vi "Test 4_5.vi"(8 "error in (no error)":errorcluster, 11 "Test Case In":refnum<class "Tests.lvclass">) -> (0 "error out":errorcluster, 3 "Test Case Out":refnum<class "Tests.lvclass">)   [LabVIEW 2021, in "Tests.lvclass"]
uses:
  Tests.lvclass
  C:/Program Files (x86)/National Instruments/LabVIEW 2021/vi.lib/Astemes/LUnit/Test Case.lvclass
  <vilib>/Astemes/LUnit/Test Case.lvclass/Test Case.ctl
  4993e8ee-a06a-463a-9684-69129f64d5ce.vi
  <vilib>/Astemes/LUnit/Append Pass Result.vi
  <vilib>/Astemes/LUnit/Append Fail Result.vi
  <vilib>/Astemes/LUnit/Describe Comparison.vi
  <vilib>/Astemes/LUnit/Compare Variants.vi
  <vilib>/Astemes/LUnit/Variant to string.vi
  <vilib>/Utility/Data Type/Get Type Information.vi
  <vilib>/Utility/LVClass/Get LV Class Name.vi
  Proto/Board.lvclass
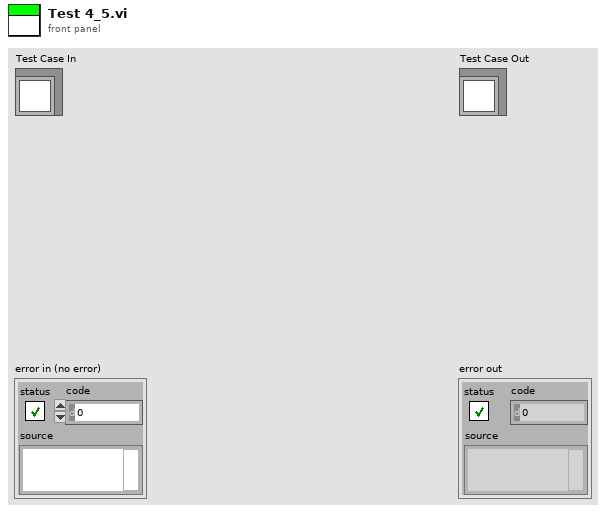
[diagram p1: front panel]
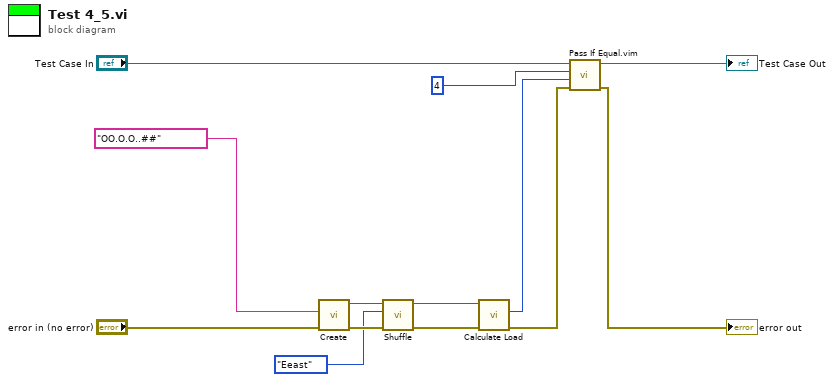
[diagram p0: block diagram]
diagram:
  n1 = call "Create.vi"("error in (no error)"="error in (no error)", "Input"="OO.O.O..##") -> ("error out"=w9:errorcluster, "Proto"=w8:refnum<class "Board.lvclass">)  [unwired: 8 in]
  n2 = call "Shuffle.vi"("error in (no error)"=w9, "North"=enum16{"North", "Eeast", "South", "West"}."Eeast", "Proto in"=w8) -> ("error out"=w6:errorcluster, "Proto out"=w4:refnum<class "Board.lvclass">)  [unwired: 7 in]
  n3 = call "Calculate Load.vi"("error in (no error)"=w6, "Proto in"=w4) -> ("error out"=w5:errorcluster, "Load"=w3:u64)  [unwired: 7 in, 1 out]
  n4 = call "Pass If Equal.vim"("error in (no error)"=w5, "Actual"=w3, "Expected"=u64 4 ("Load"), "LUnit Test Case In"="Test Case In") -> ("error out"=→"error out":errorcluster, "LUnit Test Case Out"=→"Test Case Out":refnum<class "Tests.lvclass">)  [unwired: 6 in]
